vi "ndipolaris Reset.vi"(8 "error in (no error)":errorcluster, 11 "VISA resource name":refnum<visa-resource-name>) -> (0 "error out":errorcluster, 3 "VISA resource out":refnum<visa-resource-name>)   [LabVIEW 2013]
doc: "This VI resets the I/O interface with the instrument with a serial break, putting the instrument in a known state. There is a 5 second delay after the serial break is issued before communication can be resumed."
uses:
  <vilib>/Instr/_visa.llb/VISA Serial Break (Instr).vi
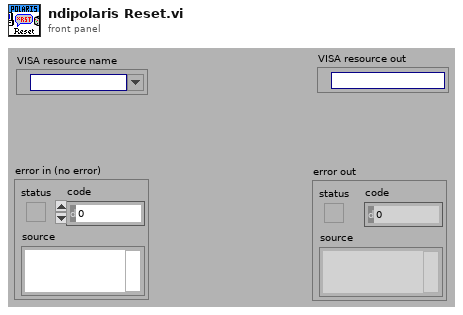
[diagram p1: front panel]
types:
  T1 = cluster{"Baud Rate (9600)":u32, "Flow Control (0:None)":u16, "Parity":u16, "Data Bits":u16, "Stop Bits":u16}
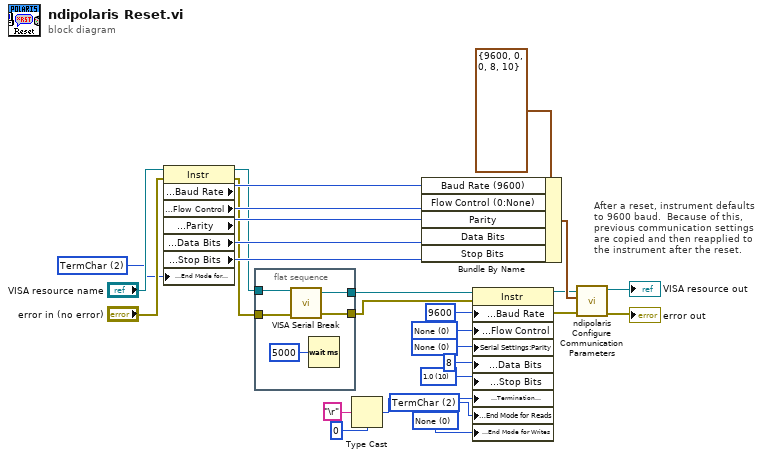
[diagram p0: block diagram]
diagram:
  w1 = u16 0 items=["None", "Last Bit", "TermChar", "Break"] ("Serial Settings:Serial End Mode for Writes")
  w2 = u16 2 items=["None", "Last Bit", "TermChar"] ("Serial Settings:Serial End Mode for Reads")
  w6 = u16 2 items=["None", "Last Bit", "TermChar"] ("Serial Settings:Serial End Mode for Reads")
  w7 = u16 10 items=["1.0"=10, "1.5"=15, "2.0"=20] ("Serial Settings:Serial Stop Bits")
  w9 = u16 0 items=["None", "Odd", "Even", "Mark", "Space"] ("Serial Settings:Serial Parity")
  w10 = u16 0 items=["None", "XON/XOFF", "RTS/CTS", "XON/XOFF & RTS/CTS", "DTR/DSR", "XON/XOFF & DTR/DSR"] ("Serial Settings:Serial Flow Control")
  # "After a reset, instrument defaults\nto 9600 baud.  Because of this,\nprevious communication settings\nare copied and then reapplied to\nthe instrument after the reset."
  n1 = property class="Instr"(reference="VISA resource name", error in="error in (no error)", "Serial Settings:End Mode for Reads"=w6) -> (reference out=w16:refnum<visa-resource-name>, error out=w17:errorcluster, "Serial Settings:Baud Rate"=w23:u32, "Serial Settings:Flow Control"=w22:u16, "Serial Settings:Parity"=w21:u16, "Serial Settings:Data Bits"=w20:u16, "Serial Settings:Stop Bits"=w19:u16)
  n2 = flat-sequence {
    tunnel: w16 -> [w33]
    tunnel: w17 -> [w32]
    tunnel: [w31] -> w15
    tunnel: [w30] -> w14
    frame #0 {
      n3 = call-poly <vilib>:"VISA Serial Break.vi"("error in (no error)"=w32, "VISA resource name"=w33) -> ("error out"=w31:errorcluster, "VISA resource name out"=w30:refnum<visa-resource-name>)  [unwired: 2 in]
      n4 = Wait (ms)(milliseconds to wait=u32 5000) -> ()  [unwired: 1 out]
    }
  }
  n5 = Type Cast(type=u8 0, x="\r") -> (*(type *) &x=w3:u8)
  n6 = Bundle By Name(cluster=T1 {"Baud Rate (9600)"=9600, "Flow Control (0:None)"=0, "Parity"=0, "Data Bits"=8, "Stop Bits"=10} ("Serial Configuration"), "Baud Rate (9600)"=w23, "Flow Control (0:None)"=w22, "Parity"=w21, "Data Bits"=w20, "Stop Bits"=w19) -> (w24:T1)
  n7 = property class="Instr"(reference=w14, error in=w15, "Serial Settings:Baud Rate"=u32 9600 ("Serial Settings:Serial Baud Rate"), "Serial Settings:Flow Control"=w10, "Serial Settings:Parity"=w9, "Serial Settings:Data Bits"=u16 8 ("Serial Settings:Serial Data Bits"), "Serial Settings:Stop Bits"=w7, "Message Based Settings:Termination Character"=w3, "Serial Settings:End Mode for Reads"=w2, "Serial Settings:End Mode for Writes"=w1) -> (reference out=w13:refnum<visa-resource-name>, error out=w12:errorcluster)
  n8 = call <instrlib>:"ndipolaris Configure Communication Parameters.vi"("error in (no error)"=w12, "Serial Configuration"=w24, "VISA resource name"=w13) -> ("error out"=→"error out":errorcluster, "VISA resource out"=→"VISA resource out":refnum<visa-resource-name>)  [unwired: 7 in]
